vi "GitAdd.vi"(8 "error in (no error)":errorcluster, 9 "File":path=path "", 11 "Git exec":string="git") -> (0 "error out":errorcluster, 1 "File out":path, 2 "Response":string, 3 "Git exec out":string="git")   [LabVIEW 2013]
uses:
  GitCmd.vi
  <vilib>/dlg_ctls.llb/Space Constant.vi
  GitUtils/PathtoDirPath.vi
  <vilib>/Platform/system.llb/System Exec.vi
  <vilib>/Utility/error.llb/Error Cluster From Error Code.vi
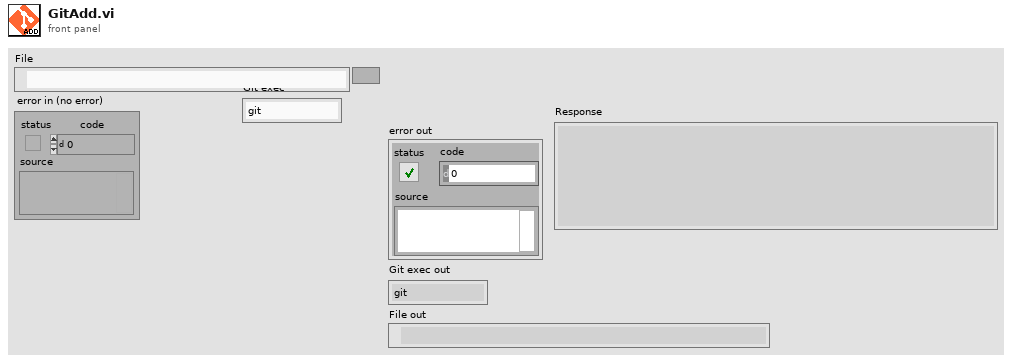
[diagram p1: front panel]
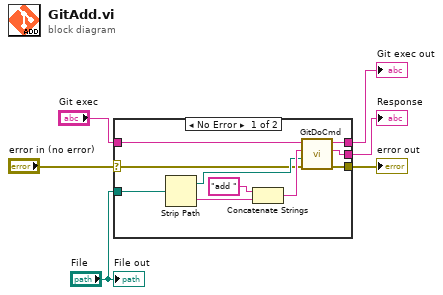
[diagram p0: block diagram]
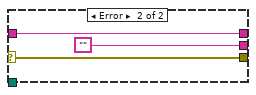
[diagram p2: hidden frame]
diagram:
  n1 = case shown="No Error" "error in (no error)" {
    selector: "error in (no error)" -> [w8 w18]
    tunnel: "Git exec" -> [w13 w17]
    tunnel: "File" -> [w15 _]
    tunnel: [w10 ""] -> w4
    tunnel: [w7 w18] -> w3
    tunnel: [w11 w17] -> w1
    frame No Error {
      n2 = Strip Path(path=w15) -> (stripped path=w9:path, name=w14:string)
      n3 = Concatenate Strings("add " ("string"), w14) -> (w12:string)
      n4 = call "GitDoCmd.vi"("error in (no error)"=w8, "Working Path"=w9, "Git command"=w12, "Git exec"=w13) -> ("error out"=w7:errorcluster, "Returned stdout"=w10:string, "Git exec out"=w11:string)  [unwired: 3 in, 1 out]
    }
    frame Error {
    }
  }
  "Response" <- w4
  "error out" <- w3
  "Git exec out" <- w1
  "File out" <- "File"
